vi "csmdoc_export_VI_description.vi"(8 "error in (no error)":errorcluster, 11 "Path":path) -> (0 "error out":errorcluster, 3 "concatenated string":string)   [LabVIEW 2017]
uses:
  Communicable State Machine.lvlib
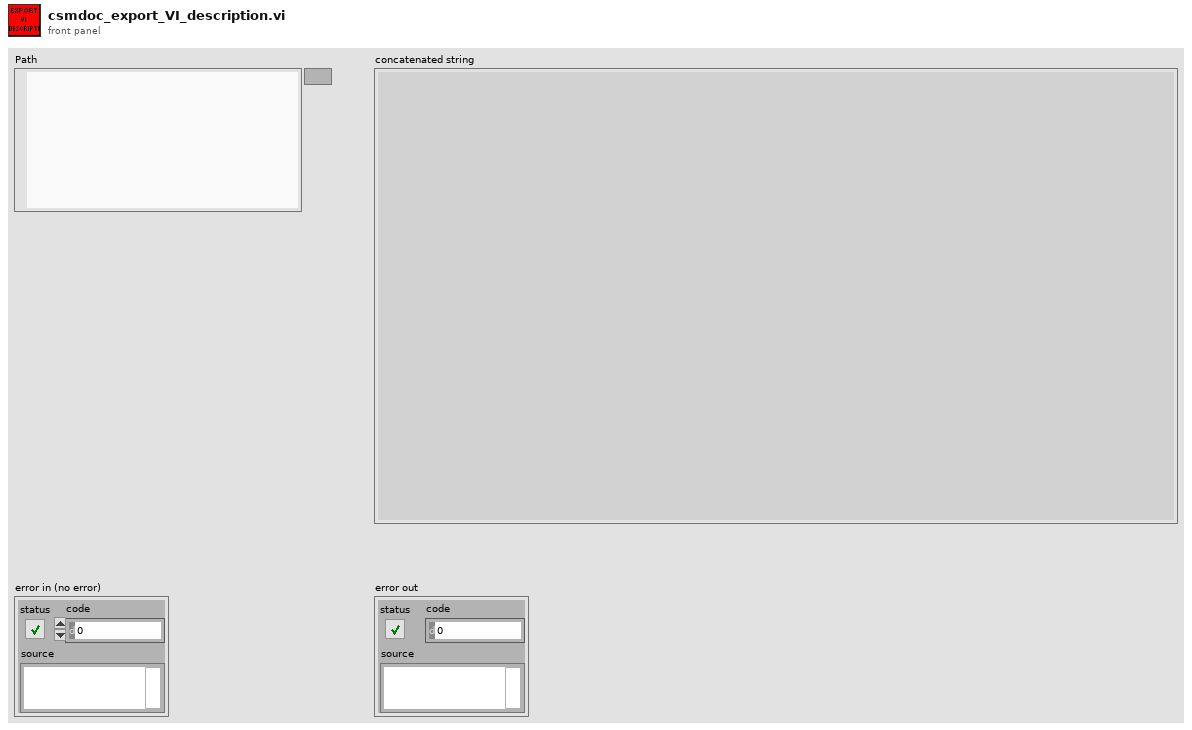
[diagram p1: front panel]
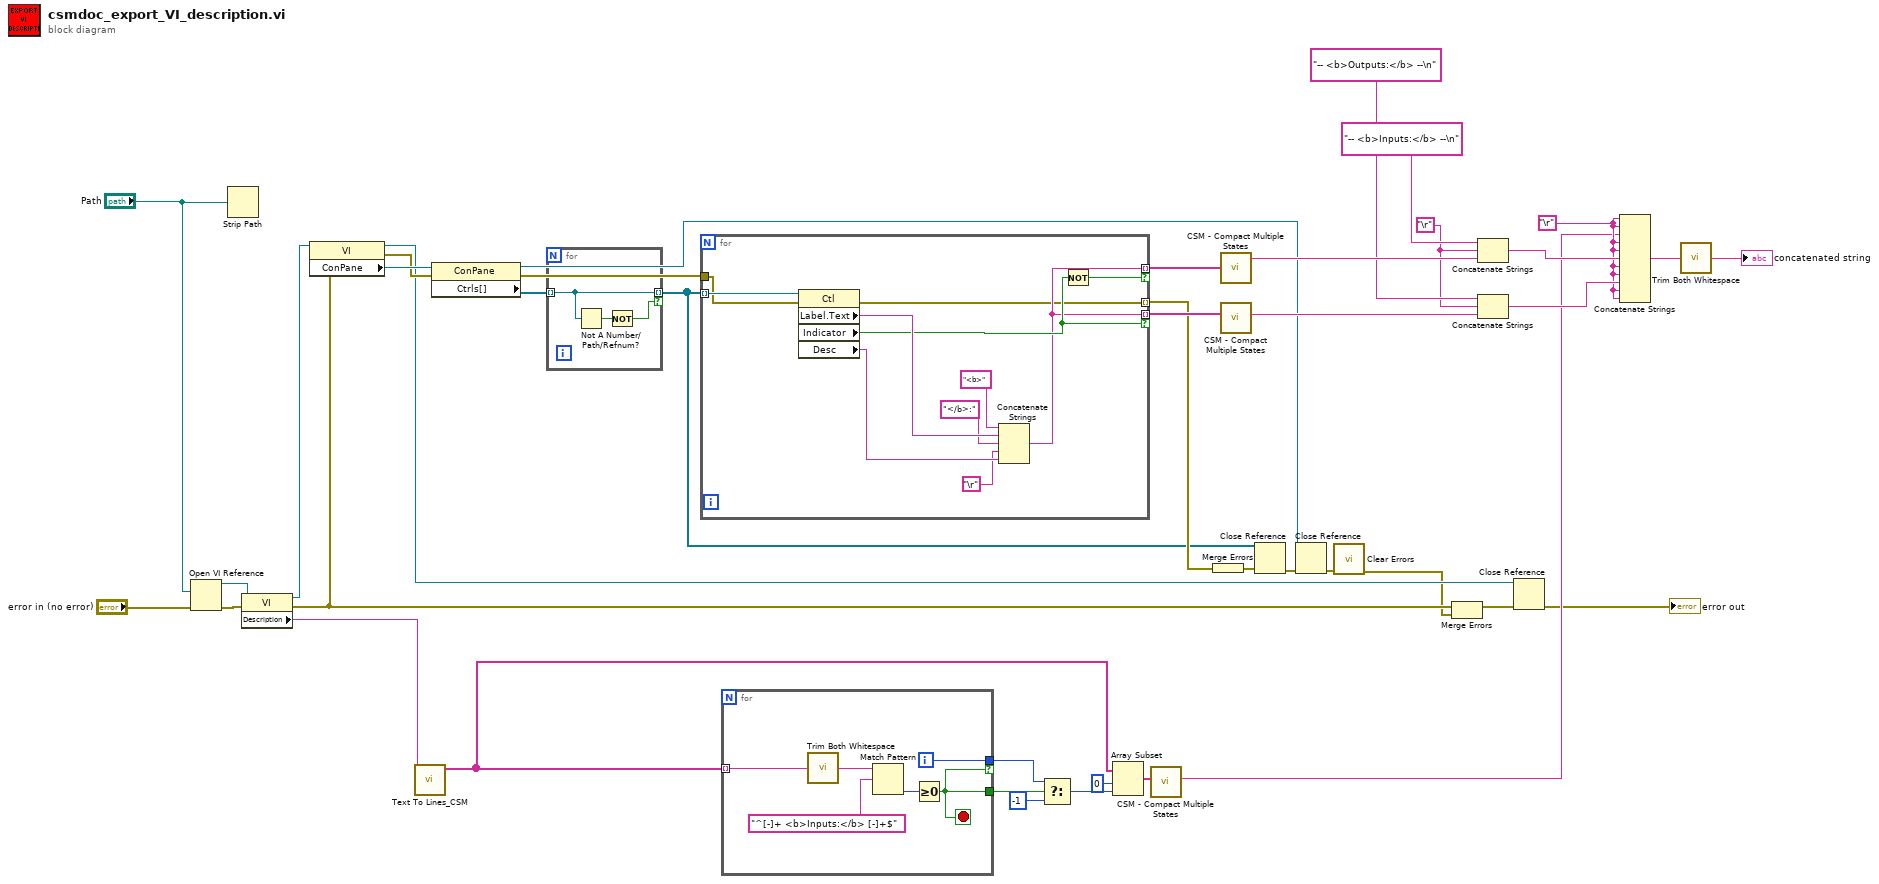
[diagram p0: block diagram]
diagram:
  w21 = "\r"
  w20 = "\r"
  n1 = Open VI Reference(vi path="Path", error in (no error)="error in (no error)") -> (vi reference=w40:refnum<vi>, error out=w41:errorcluster)  [unwired: 4 in]
  n2 = Strip Path(path="Path") -> ()  [unwired: 2 out]
  n3 = property class="VI"(reference=w40, error in=w41) -> (reference out=w38:refnum<vi>, error out=w18:errorcluster, "Description"=w39:string)
  n4 = property class="VI"(reference=w38, error in=w18) -> (reference out=w22:refnum<vi>, error out=w28:errorcluster, "ConPane"=w37:refnum<vi>)
  n5 = call "Text To Lines_CSM.vi"("string"=w39) -> ("Lines"=w6:string[])  [unwired: 9 in, 1 out]
  n6 = property class="ConPane"(reference=w37, error in=w28) -> (reference out=w23:refnum<vi>, error out=w26:errorcluster, "Ctrls[]"=w2:refnum<vi>[])
  n7 = for {
    tunnel: w2 -> [w44] mode=indexing
    tunnel: [w44] -> w1 mode=indexing if=w42
    n8 = Not A Number/Path/Refnum?(number/path/refnum=w44) -> (NaN/Path/Refnum?=w43:bool)
    n9 = Not(x=w43) -> (.not. x?=w42:bool)
  }
  n10 = for {
    tunnel: w1 -> [w55] mode=indexing
    tunnel: [w51] -> w36 mode=indexing if=w52
    tunnel: [w51] -> w35 mode=indexing if=w53
    tunnel: w26 -> [w49]
    tunnel: [w48] -> w25 mode=indexing
    n11 = property class="Ctl"(reference=w55, error in=w49) -> (error out=w48:errorcluster, "Label.Text"=w54:string, "Indicator"=w53:bool, "Desc"=w46:string)  [unwired: 1 out]
    n12 = Concatenate Strings("<b>" ("string"), w54, "</b>:" ("string"), "\r", w46) -> (w51:string)
    n13 = Not(x=w53) -> (.not. x?=w52:bool)
  }
  n14 = for {
    tunnel: w6 -> [w61] mode=indexing
    tunnel: [w57] -> w9 if=w56
    tunnel: [w56] -> w10
    i -> [w57]
    stop <- w56 stop-if-true
    n15 = call "Trim Both Whitespace.vi"("string"=w61) -> ("trimmed string"=w59:string)  [unwired: 1 in]
    n16 = Match Pattern(string=w59, regular expression="^[-]+ <b>Inputs:</b> [-]+$") -> (offset past match=w58:i32)  [unwired: 1 in, 3 out]
    n17 = Greater Or Equal To 0?(x=w58) -> (x >= 0?=w56:bool)
  }
  n18 = Select(t=w9, s=w10, f=-1) -> (s? t:f=w7:i32)
  n19 = Array Subset(array=w6, index=0, length=w7) -> (w4:string[])
  n20 = call "CSM - Compact Multiple States.vi"("Multiple States"=w4) -> ("States"=w19:string)  [unwired: 9 in]
  n21 = Merge Errors(w25) -> (w24:errorcluster)
  n22 = call "CSM - Compact Multiple States.vi"("Multiple States"=w36) -> ("States"=w33:string)  [unwired: 9 in]
  n23 = call "CSM - Compact Multiple States.vi"("Multiple States"=w35) -> ("States"=w34:string)  [unwired: 9 in]
  n24 = Close Reference(reference=w1, error in (no error)=w24) -> (error out=w27:errorcluster)
  n25 = Close Reference(reference=w23, error in (no error)=w27) -> (error out=w17:errorcluster)
  n26 = call <vilib>:"Clear Errors.vi"("error in (no error)"=w17) -> ("error out"=w11:errorcluster)  [unwired: 5 in, 1 out]
  n27 = Merge Errors(w18, w11) -> (w16:errorcluster)
  n28 = Concatenate Strings("-- <b>Inputs:</b> --\n" ("string"), w21, w33) -> (w30:string)
  n29 = Concatenate Strings("-- <b>Outputs:</b> --\n" ("string"), w21, w34) -> (w29:string)
  n30 = Close Reference(reference=w22, error in (no error)=w16) -> (error out=→"error out":errorcluster)
  n31 = Concatenate Strings(w20, w20, w19, w20, w20, w30, w20, w20, w29, w20, w20) -> (w14:string)
  n32 = call "Trim Both Whitespace.vi"("string"=w14) -> ("trimmed string"=→"concatenated string":string)  [unwired: 1 in]
